vi "Read TDATA Core.vi"(11 "niInstr AXI4-Stream Reader FXP64x4 v1 FPGA in":refnum<class "niInstr AXI4-Stream Reader FXP64x4 v1 FPGA.lvclass">) -> (2 "tdata value":bool[](array[boolean]), 3 "niInstr AXI4-Stream Reader FXP64x4 v1 FPGA out":refnum<class "niInstr AXI4-Stream Reader FXP64x4 v1 FPGA.lvclass">)   [LabVIEW 2015, in "niInstr AXI4-Stream Reader FXP64x4 v1 FPGA.lvclass"]
doc: "<B>Output Parameters</B>\n\n<B>tdata value</B> is the value in the returned TDATA."
uses:
  <instrlib>/_niInstr/CLIP Adapters/v1/FPGA/AXI4-Stream/Reader FXP64x4/niInstr AXI4-Stream Reader FXP64x4 v1 FPGA.lvclass
  <instrlib>/_niInstr/CLIP Adapters/v1/FPGA/AXI4-Stream/Reader FXP64x4/niInstr AXI4-Stream Reader FXP64x4 v1 FPGA.lvclass/niInstr AXI4-Stream Reader FXP64x4 v1 FPGA.ctl
  <instrlib>/_niInstr/Data Formatting/v1/FPGA/Private/Convert/U64 array to Boolean Array.vi
  <vilib>/rvi/eio/common/nirviEmuTemplateMethod_errors.vi
  <vilib>/eio/EIONode/EIONode.xnode
  <instrlib>/_niInstr/Data Formatting/v1/FPGA/niInstr Data Formatting v1 FPGA.lvlib
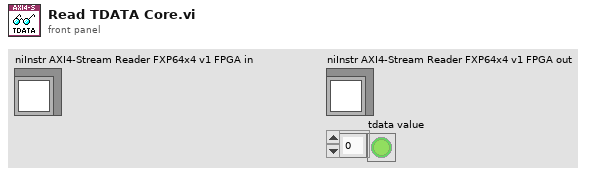
[diagram p1: front panel]
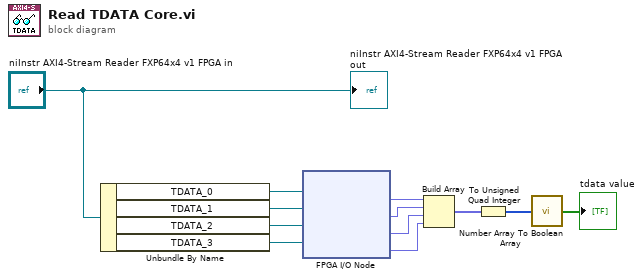
[diagram p0: block diagram]
diagram:
  n1 = Unbundle By Name("niInstr AXI4-Stream Reader FXP64x4 v1 FPGA in") -> ("TDATA_0"=w11:refnum<k21>, "TDATA_1"=w10:refnum<k21>, "TDATA_2"=w9:refnum<k21>, "TDATA_3"=w8:refnum<k21>)
  n2 = xnode "FPGA I/O Node"("FPGA I/O In"=w11, "FPGA I/O In"=w10, "FPGA I/O In"=w9, "FPGA I/O In"=w8) -> ("I/O Item"=w7:fxp<+,64,64>, "I/O Item"=w6:fxp<+,64,64>, "I/O Item"=w5:fxp<+,64,64>, "I/O Item"=w4:fxp<+,64,64>)  [unwired: 4 out]
  n3 = Build Array(w7, w6, w5, w4) -> (w2:fxp<+,64,64>[])
  n4 = To Unsigned Quad Integer(1:w2) -> (0:w1:u64[])
  n5 = call-poly <instrlib>:"Number Array To Boolean Array.vi"("data in"=w1) -> ("data out"=→"tdata value":bool[])  [unwired: 14 in]
  "niInstr AXI4-Stream Reader FXP64x4 v1 FPGA out" <- "niInstr AXI4-Stream Reader FXP64x4 v1 FPGA in"
